vi "Analog Voltage On.vi"(8 "error in (no error)":errorcluster, 11 "Voltage":sgl) -> (3 "Queue Out":T1)   [LabVIEW 2023, in "FPGA.lvlib"]
doc: "VI activate the analog output voltage of the system"
uses:
  FPGA.lvlib
  Internal Communication/Controls/Queue.ctl
panel:
  out "error out":errorcluster
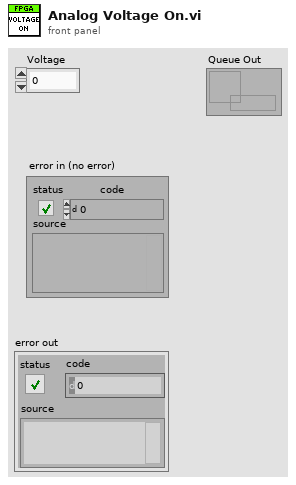
[diagram p1: front panel]
types:
  T1 = typedef "Queue.ctl" = refnum<queue>
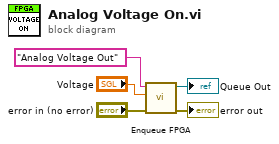
[diagram p0: block diagram]
diagram:
  n1 = call "Enqueue FPGA.vi"("error in (no error)"="error in (no error)", "Data"="Voltage", "Command"="Analog Voltage Out") -> ("error out"=→"error out":errorcluster, "Queue Out"=→"Queue Out":T1)  [unwired: 7 in]
